vi "camera-make_write-frame.vi"(10 "Data":string, 11 "Address":string) -> (3 "Serial String":string)   [LabVIEW 2012]
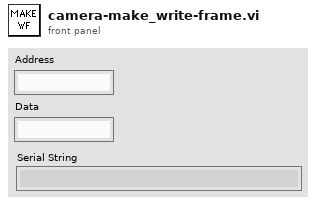
[diagram p1: front panel]
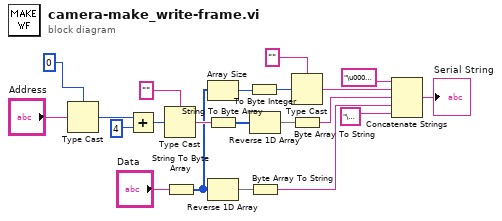
[diagram p0: block diagram]
diagram:
  n1 = Type Cast(type=u32 0 ("y"), x="Address") -> (*(type *) &x=w16:u32)
  n2 = Add(x=w16, y=u32 4) -> (x+y=w15:u32)
  n3 = Type Cast(type="", x=w15) -> (*(type *) &x=w11:string)
  n4 = String To Byte Array(string="Data") -> (unsigned byte array=w4:u8[])
  n5 = Array Size(array=w4) -> (size(s)=w2:i32)
  n6 = String To Byte Array(string=w11) -> (unsigned byte array=w13:u8[])
  n7 = Reverse 1D Array(array=w4) -> (reversed array=w20:u8[])
  n8 = To Byte Integer(number=w2) -> (8bit integer=w1:i8)
  n9 = Reverse 1D Array(array=w13) -> (reversed array=w12:u8[])
  n10 = Byte Array To String(unsigned byte array=w20) -> (string=w9:string)
  n11 = Type Cast(type="", x=w1) -> (*(type *) &x=w3:string)
  n12 = Byte Array To String(unsigned byte array=w12) -> (string=w10:string)
  n13 = Concatenate Strings("\u0001\u0001", w3, w10, w9, "\u0003") -> (→"Serial String":string)
